vi "Close File+.vi"(0 "error in (no error)":errorcluster caption="Fehler (Eingang, kein Fehler)", 1 "close when? (now:T)":bool=TRUE caption="Wann schließen? (jetzt:T)", 4 "refnum":refnum<file> caption="RefNum") -> (3 "error out":errorcluster caption="Fehler (Ausgang)", 6 "file size (bytes)":i32 caption="Dateigröße (Byte)", 7 "refnum":refnum<file> caption="RefNum")   [LabVIEW 2009]
doc: "Schließt die Datei, bei aufruf des Befehls zum Schließen oder wenn ein Fehler auftritt und gibt die Dateigröße zurück.\n\nRefnum ist die Referenz der offenen Datei.\n\nWann schließen? Auf TRUE (Voreinstellung), wenn Sie die Datei schließen möchten, wenn das VI aufgerufen wird . Auf FALSE, wenn Sie die Datei nur dann schließen möchten, wenn ein Fehler auftritt. Dieser Eingang ist hilfreich, wenn Sie das VI in einer Schleife verwenden und die Datei erst im letzten Schleifendurchlauf oder wenn ein Fehler auftritt schließen möchten. In diesem Fall muss \"Wann schließen?\" gesetzt werden. im letzten Durchlauf auf TRUE gesetzt werden und die Schleife verlassen werden. \n\nDateigröße ist die Dateigröße in Byte zu dem Zeitpunkt zu dem die Datei geschlossen wird; sonst ist der Wert 0.\n\nFehlereingang ist ein Cluster mit 3 Elementen (Fehler?, Code, und Quelle) welches die Fehler des Speichervorganges anzeigt. Das VI kann nur dann normal ausgeführt werden, wenn kein Eingangsfehler vorliegt; sonst wird der vorher aufgetretene Fehler weitergeleitet. Fehler? ist TRUE, wenn ein Fehler aufgetreten ist; die Voreinstellung ist FALSE. Code ist der Fehlercode; die Voreinstellung ist 0. Quelle ist in den meisten Fällen der Name des VIs oder der Funktion in welcher der Fehler aufgetreten ist; die Voreinstellung ist ein leerer String. \n\nRefNum (Kopie) leitet die Referenznummer weiter.\n\nFehlerausgang ist ein Cluster mit 3 Elementen (Fehler?, Code, und Quelle) welches den Fehlerstatus nach Ablauf des VIs beschreibt. Wenn kein Eingangsfehler auftrat, wird das VI normal ausgeführt und der Fehlerausgang enthält den Fehlerstatus dieses VIs; wenn ein Eingangsfehler auftrat wird diesen an den Fehlerausgang weitergegeben."
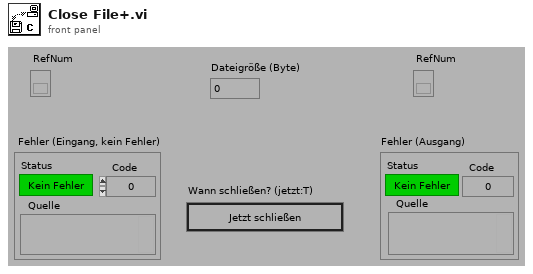
[diagram p1: front panel]
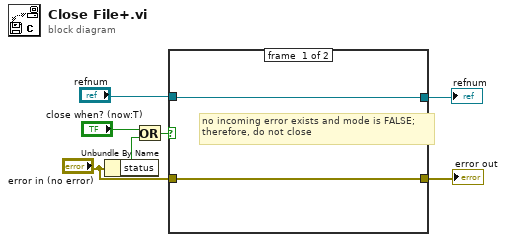
[diagram p0: block diagram]
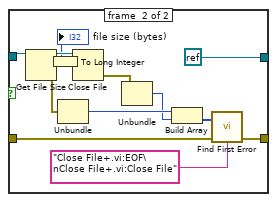
[diagram p2: hidden frame]
diagram:
  n1 = Unbundle By Name("error in (no error)") -> ("status"=w1:bool)
  n2 = Or(x="close when? (now:T)", y=w1) -> (x .or. y?=w6:bool)
  n3 = case shown="True" w6 {
    tunnel: [w9 w13] -> w5
    tunnel: "error in (no error)" -> [w9 w16]
    tunnel: [w8 refnum<k0> refnum] -> w4
    tunnel: "refnum" -> [w8 w20]
    frame #0 {
      # "no incoming error exists and mode is FALSE;\ntherefore, do not close"
    }
    frame #1 {
      n4 = Get File Size(file=w20) -> (refnum out=w21:refnum<file>, size (in bytes)=w10:i64, 0:w18:errorcluster)  [unwired: 1 in]
      n5 = To Long Integer(number=w10) -> (32bit integer=→"file size (bytes)":i32)
      n6 = Unbundle(w18) -> ("code"=w12:i32)  [unwired: 2 out]
      n7 = Close File(refnum=w21) -> (error out=w17:errorcluster)  [unwired: 1 in, 1 out]
      n8 = Unbundle(w17) -> ("code"=w11:i32)  [unwired: 2 out]
      n9 = Build Array(w12, w11) -> (w15:i32[])
      n10 = call "Find First Error.vi"("error in (no error)"=w16, "source messages"="Close File+.vi:EOF\nClose File+.vi:Close File", "error codes"=w15) -> ("error out"=w13:errorcluster)  [unwired: 1 in, 1 out]
    }
  }
  "error out" <- w5
  "refnum" <- w4
